vi "decodeStream.vi"(8 "error in (no error)":errorcluster, 9 "Begin Index":i32, 10 "Byte Data In":u8[](array[numeric])) -> (0 "error out":errorcluster, 1 "End Index":i32, 2 "Byte Data Out":u8[](array[numeric]), 3 "tBSONDocument out":refnum<class "tBSONDocument.lvclass">)   [LabVIEW 2013, in "BSON.lvlib" / "tBSONDocument.lvclass"]
doc: "Starting at Begin Index, extracts a document from a BSON byte stream."
uses:
  tBSONDocument.lvclass
  status.ctl
  tBSONElement/tBSONElement.lvclass
  BSONElements/tBSONDouble/tBSONDouble.lvclass
  BSONElements/tBSONString/tBSONString.lvclass
  BSONElements/tBSONDocumentElement/tBSONDocumentElement.lvclass
  BSONElements/tBSONArray/tBSONArray.lvclass
  BSONElements/tBSONBinary/tBSONBinary.lvclass
  BSONElements/tBSONObjectID/tBSONObjectID.lvclass
  BSONElements/tBSONBoolean/tBSONBoolean.lvclass
  BSONElements/tBSONTimestamp/tBSONTimestamp.lvclass
  BSONElements/tBSONNull/tBSONNull.lvclass
  BSONElements/tBSONRegEx/tBSONRegEx.lvclass
  BSONElements/tBSONJavaScript/tBSONJavaScript.lvclass
  BSONElements/tBSONJavaScriptWithScope/tBSONJavaScriptWithScope.lvclass
  BSONElements/tBSON_I32/tBSON_I32.lvclass
  BSONElements/tBSON_I64/tBSON_I64.lvclass
  BSON.lvlib
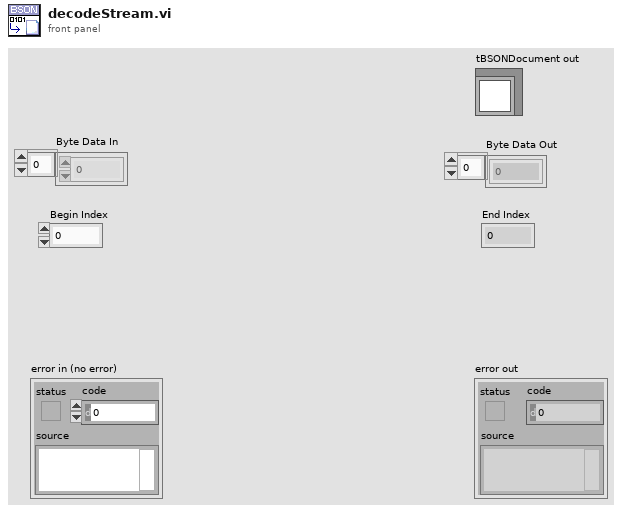
[diagram p1: front panel]
types:
  T1 = typedef "BSON.lvlib/status.ctl" = enum16{"Stream Corrupted or Ended Abruptly", "Incorrect Type In Stream", "ObjectID Invalid", "Method Not Implemented", "Invalid Name", "Invalid URI", "AutoReconnect", "Operation Failed", "Incorrectly Configured", "Cursor Not Found", "Timeout", "Invalid Type", "Empty Name", "Duplicate Name", "MD5Incorrect"}
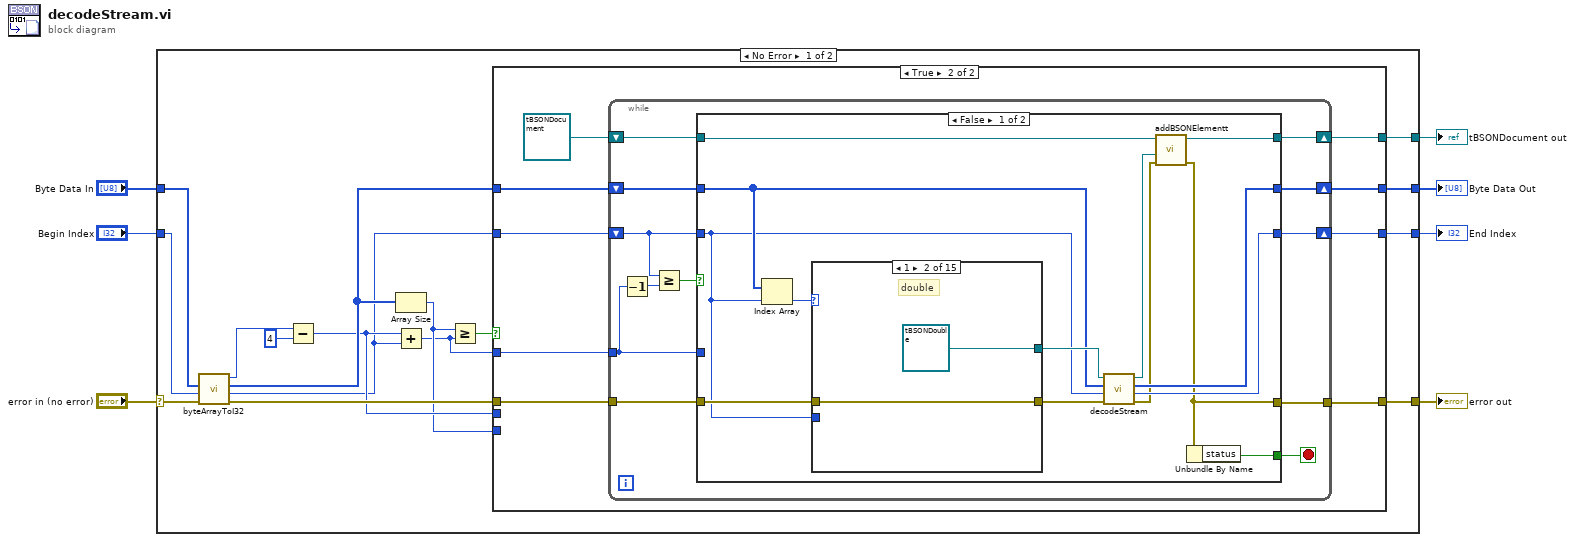
[diagram p0: block diagram]
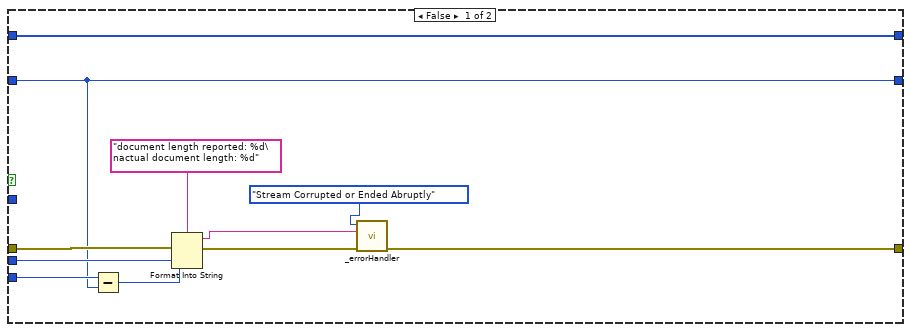
[diagram p2: hidden frame]
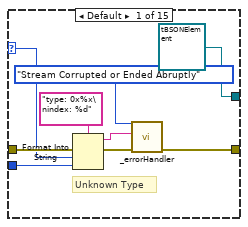
[diagram p3: hidden frame]
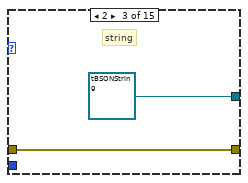
[diagram p4: hidden frame]
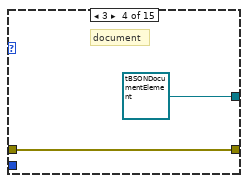
[diagram p5: hidden frame]
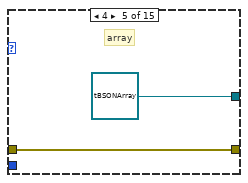
[diagram p6: hidden frame]
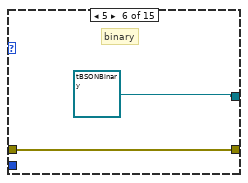
[diagram p7: hidden frame]
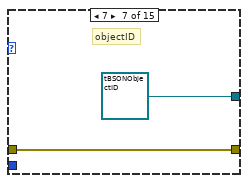
[diagram p8: hidden frame]
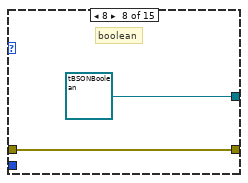
[diagram p9: hidden frame]
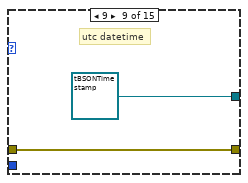
[diagram p10: hidden frame]
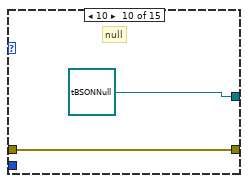
[diagram p11: hidden frame]
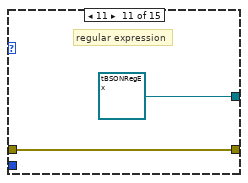
[diagram p12: hidden frame]
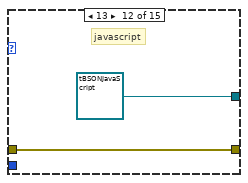
[diagram p13: hidden frame]
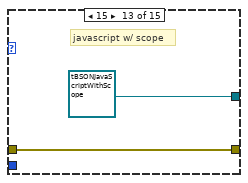
[diagram p14: hidden frame]
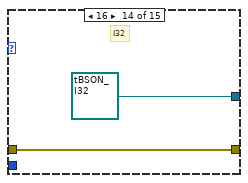
[diagram p15: hidden frame]
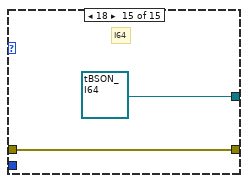
[diagram p16: hidden frame]
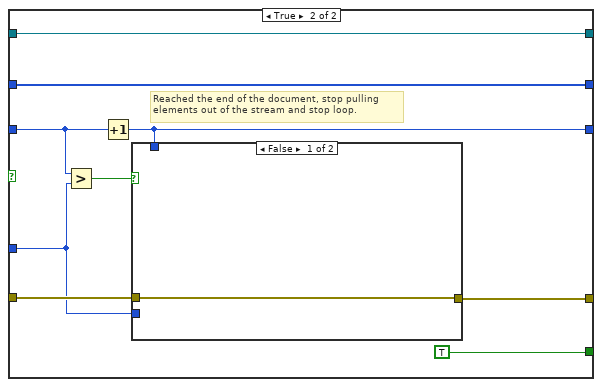
[diagram p17: hidden frame]
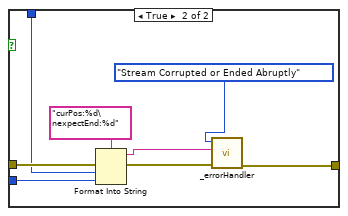
[diagram p18: hidden frame]
diagram:
  n1 = case shown="No Error" "error in (no error)" {
    selector: "error in (no error)" -> [w23 w127]
    tunnel: [w14 w127] -> w6
    tunnel: [w15 _] -> w5
    tunnel: "Byte Data In" -> [w22 w126]
    tunnel: [w16 w126] -> w3
    tunnel: "Begin Index" -> [w21 w125]
    tunnel: [w17 w125] -> w1
    frame No Error {
      n2 = call "byteArrayToI32.vi"("error in (no error)"=w23, "StartIndex"=w21, "ByteArrayIn"=w22) -> ("error out"=w18:errorcluster, "EndIndex"=w8:i32, "ByteArrayOut"=w13:u8[], "I32"=w20:i32)  [unwired: 5 in]
      n3 = Subtract(x=w20, y=4) -> (x-y=w11:i32)
      n4 = Array Size(array=w13) -> (size(s)=w10:i32)
      n5 = Add(x=w11, y=w8) -> (x+y=w9:i32)
      n6 = Greater Or Equal?(x=w10, y=w9) -> (x >= y?=w12:bool)
      n7 = case shown="True" w12 {
        tunnel: w18 -> [w31 w40]
        tunnel: w11 -> [w29 _]
        tunnel: w8 -> [w24 w42]
        tunnel: [w24 w36] -> w17
        tunnel: w13 -> [w28 w43]
        tunnel: [w28 w37] -> w16
        tunnel: [_ w38] -> w15
        tunnel: [w27 w39] -> w14
        tunnel: w9 -> [_ w41]
        tunnel: w10 -> [w25 _]
        frame False {
          n8 = Subtract(x=w25, y=w24) -> (x-y=w26:i32)
          n9 = Format Into String(format string="document length reported: %d\nactual document length: %d", error in=w31, w29, w26) -> (resulting string=w34:string, error out=w33:errorcluster)  [unwired: 1 in]
          n10 = call "_errorHandler.vi"("error in (no error)"=w33, "Additional Text"=w34, "Error Type"=status."Stream Corrupted or Ended Abruptly") -> ("error out"=w27:errorcluster)  [unwired: 8 in]
        }
        frame True {
          n11 = while {
            shift-right: [w51] -> w38
            shift-left: refnum<class "tBSONDocument.lvclass"> refnum ("lvMongoDriver.lvlib:BSON.lvlib:tBSONDocument.lvclass") -> [w54]
            shift-right: [w52] -> w37
            shift-left: w43 -> [w55]
            shift-right: [w53] -> w36
            shift-left: w42 -> [w46]
            tunnel: w41 -> [w45]
            tunnel: w40 -> [w49]
            tunnel: [w48] -> w39
            stop <- w50 stop-if-true
            n12 = Decrement(x=w45) -> (x-1=w44:i32)
            n13 = Greater Or Equal?(x=w46, y=w44) -> (x >= y?=w47:bool)
            n14 = case shown="False" w47 {
              tunnel: w46 -> [w56 w108]
              tunnel: w55 -> [w64 w115]
              tunnel: w54 -> [w61 w114]
              tunnel: [w62 w107] -> w53
              tunnel: [w63 w115] -> w52
              tunnel: [w60 w114] -> w51
              tunnel: [w68 TRUE] -> w50
              tunnel: w49 -> [w69 w112]
              tunnel: w45 -> [_ w109]
              tunnel: [w58 w111] -> w48
              frame False {
                n15 = Index Array(array=w64, index=w56) -> (element=w67:u8)
                n16 = case shown="1" w67 {
                  selector: w67 -> [w72 _ _ _ _ _ _ _ _ _ _ _ _ _ _]
                  tunnel: w69 -> [w75 w79 w82 w83 w85 w87 w89 w91 w93 w95 w97 w99 w101 w103 w105]
                  tunnel: [w77 w79 w82 w83 w85 w87 w89 w91 w93 w95 w97 w99 w101 w103 w105] -> w66
                  tunnel: [refnum<class "tBSONElement.lvclass"> refnum ("BSON.lvlib:tBSONElement.lvclass") refnum<class "tBSONDouble.lvclass"> refnum ("BSON.lvlib:tBSONDouble.lvclass") refnum<class "tBSONString.lvclass"> refnum ("BSON.lvlib:tBSONString.lvclass") refnum<class "tBSONDocumentElement.lvclass"> refnum ("BSON.lvlib:tBSONDocumentElement.lvclass") refnum<class "tBSONArray.lvclass"> refnum ("BSON.lvlib:tBSONArray.lvclass") refnum<class "tBSONBinary.lvclass"> refnum ("BSON.lvlib:tBSONBinary.lvclass") refnum<class "tBSONObjectID.lvclass"> refnum ("BSON.lvlib:tBSONObjectID.lvclass") refnum<class "tBSONBoolean.lvclass"> refnum ("BSON.lvlib:tBSONBoolean.lvclass") refnum<class "tBSONTimestamp.lvclass"> refnum ("BSON.lvlib:tBSONTimestamp.lvclass") refnum<class "tBSONNull.lvclass"> refnum ("BSON.lvlib:tBSONNull.lvclass") refnum<class "tBSONRegEx.lvclass"> refnum ("BSON.lvlib:tBSONRegEx.lvclass") refnum<class "tBSONJavaScript.lvclass"> refnum ("BSON.lvlib:tBSONJavaScript.lvclass") refnum<class "tBSONJavaScriptWithScope.lvclass"> refnum ("BSON.lvlib:tBSONJavaScriptWithScope.lvclass") refnum<class "tBSON_I32.lvclass"> refnum ("BSON.lvlib:tBSON_I32.lvclass") refnum<class "tBSON_I64.lvclass"> refnum ("BSON.lvlib:tBSON_I64.lvclass")] -> w65
                  tunnel: w56 -> [w70 _ _ _ _ _ _ _ _ _ _ _ _ _ _]
                  frame Default {
                    # "Unknown Type"
                    n17 = Format Into String(format string="type: 0x%x\nindex: %d", error in=w75, w72, w70) -> (resulting string=w71:string, error out=w74:errorcluster)  [unwired: 1 in]
                    n18 = call "_errorHandler.vi"("error in (no error)"=w74, "Additional Text"=w71, "Error Type"=status."Stream Corrupted or Ended Abruptly") -> ("error out"=w77:errorcluster)  [unwired: 8 in]
                  }
                  frame 1 {
                    # "double"
                  }
                  frame 2 {
                    # "string"
                  }
                  frame 3 {
                    # "document"
                  }
                  frame 4 {
                    # "array"
                  }
                  frame 5 {
                    # "binary"
                  }
                  frame 7 {
                    # "objectID"
                  }
                  frame 8 {
                    # "boolean"
                  }
                  frame 9 {
                    # "utc datetime"
                  }
                  frame 10 {
                    # "null"
                  }
                  frame 11 {
                    # "regular expression"
                  }
                  frame 13 {
                    # "javascript"
                  }
                  frame 15 {
                    # "javascript w/ scope"
                  }
                  frame 16 {
                    # "I32"
                  }
                  frame 18 {
                    # "I64"
                  }
                }
                n19 = call-dynamic "decodeStream.vi"("error in (no error)"=w66, "beginIndex"=w56, "binary stream"=w64, "tBSONElement in"=w65) -> ("error out"=w59:errorcluster, "endIndex"=w62:i32, "binary stream out"=w63:u8[], "tBSONElement out"=w57:refnum<class "tBSONElement.lvclass">)  [unwired: 4 in]
                n20 = call "addBSONElementt.vi"("error in (no error)"=w59, "Element"=w57, "tBSONDocument in"=w61) -> ("error out"=w58:errorcluster, "tBSONDocument out"=w60:refnum<class "tBSONDocument.lvclass">)  [unwired: 7 in]
                n21 = Unbundle By Name(w58) -> ("status"=w68:bool)
              }
              frame True {
                # "Reached the end of the document, stop pulling\nelements out of the stream and stop loop."
                n22 = Greater?(x=w108, y=w109) -> (0:w113:bool)
                n23 = Increment(x=w108) -> (x+1=w107:i32)
                n24 = case shown="False" w113 {
                  tunnel: w112 -> [w116 w122]
                  tunnel: [w116 w124] -> w111
                  tunnel: w107 -> [_ w118]
                  tunnel: w109 -> [_ w117]
                  frame False {
                  }
                  frame True {
                    n25 = Format Into String(format string="curPos:%d\nexpectEnd:%d", error in=w122, w118, w117) -> (resulting string=w121:string, error out=w119:errorcluster)  [unwired: 1 in]
                    n26 = call "_errorHandler.vi"("error in (no error)"=w119, "Additional Text"=w121, "Error Type"=status."Stream Corrupted or Ended Abruptly") -> ("error out"=w124:errorcluster)  [unwired: 8 in]
                  }
                }
              }
            }
          }
        }
      }
    }
    frame Error {
    }
  }
  "error out" <- w6
  "tBSONDocument out" <- w5
  "Byte Data Out" <- w3
  "End Index" <- w1
